vi "Gyro control.vi"(8 "Right Turn Value":dbl, 9 "Left Turn Value":dbl, 10 "Max Power":dbl, 11 "Angle":dbl) -> (2 "Value Y":dbl, 3 "Value X":dbl)   [LabVIEW 2015]
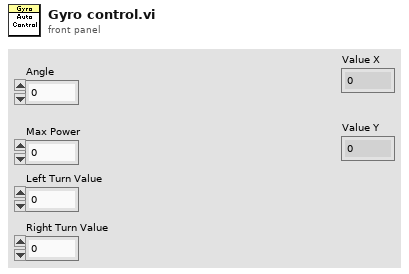
[diagram p1: front panel]
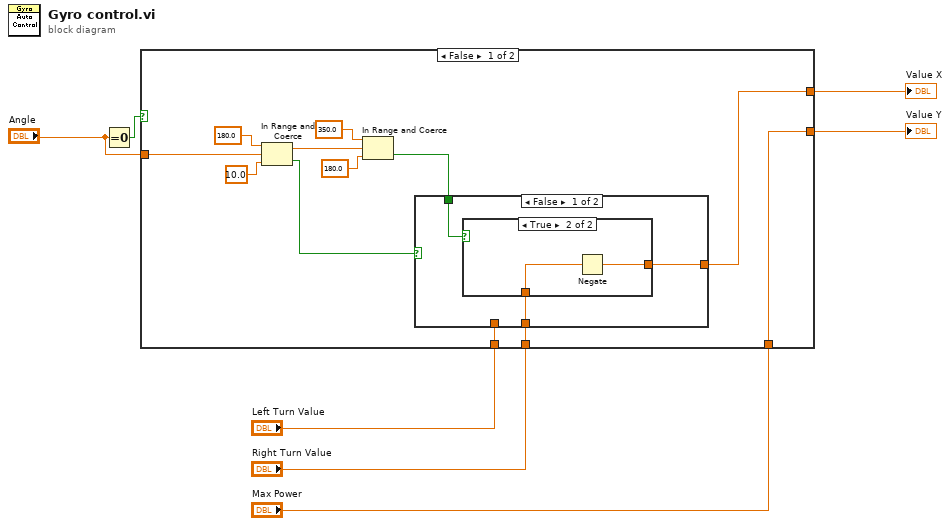
[diagram p0: block diagram]
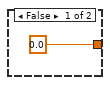
[diagram p2: hidden frame]
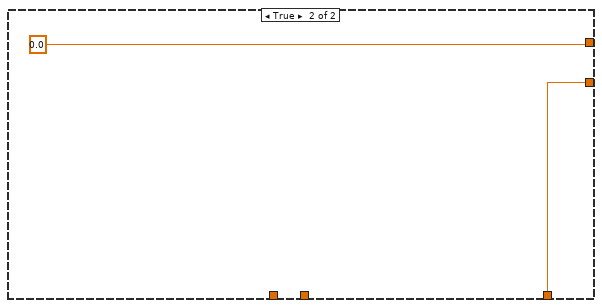
[diagram p4: hidden frame]
diagram:
  n1 = Equal To 0?(x="Angle") -> (x = 0?=w7:bool)
  n2 = case shown="False" w7 {
    tunnel: [w12 0.0] -> w6
    tunnel: [w8 w27] -> w5
    tunnel: "Angle" -> [w19 _]
    tunnel: "Left Turn Value" -> [w10 _]
    tunnel: "Right Turn Value" -> [w9 _]
    tunnel: "Max Power" -> [w8 w27]
    frame False {
      n3 = In Range and Coerce(upper limit=180.0, x=w19, lower limit=10.0) -> (coerced(x)=w14:dbl, In Range?=w13:bool)
      n4 = In Range and Coerce(upper limit=350.0, x=w14, lower limit=180.0) -> (In Range?=w11:bool)  [unwired: 1 out]
      n5 = case shown="False" w13 {
        tunnel: [w21 w26] -> w12
        tunnel: w11 -> [w22 _]
        tunnel: w10 -> [_ w26]
        tunnel: w9 -> [w20 _]
        frame False {
          n6 = case shown="True" w22 {
            tunnel: [0.0 w25] -> w21
            tunnel: w20 -> [_ w24]
            frame False {
            }
            frame True {
              n7 = Negate(x=w24) -> (-x=w25:dbl)
            }
          }
        }
        frame True {
        }
      }
    }
    frame True {
    }
  }
  "Value X" <- w6
  "Value Y" <- w5
